vi "Find Item by Tag.vi"(8 "error in (no error)":errorcluster, 10 "Tag":string, 11 "Tree Manager in":refnum<class "Tree Manager.lvclass">) -> (0 "error out":errorcluster, 1 "Found?":bool, 2 "Data Item":refnum<class "Data Item.lvclass">, 3 "Tree Manager out":refnum<class "Tree Manager.lvclass">)   [LabVIEW 2020, in "VILab.lvlib" / "Tree Manager.lvclass"]
uses:
  Tree Manager.lvclass
  Data Item/Data Item.lvclass
  Tree Manager.lvclass/Tree Manager.ctl
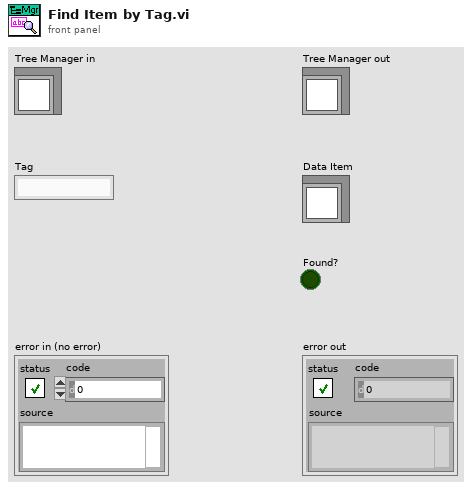
[diagram p1: front panel]
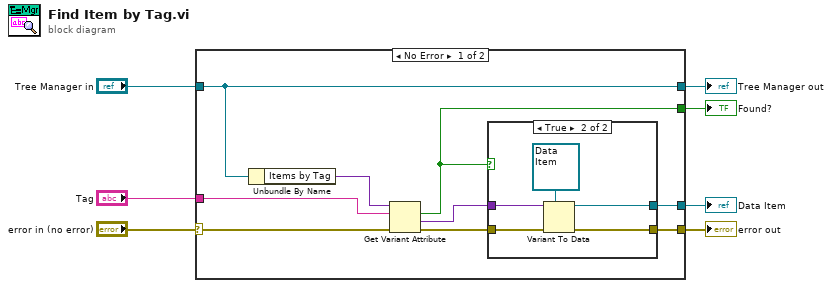
[diagram p0: block diagram]
diagram:
  n1 = case shown="No Error" "error in (no error)" {
    selector: "error in (no error)" -> [w13 w24]
    tunnel: [w10 w24] -> w6
    tunnel: [w16 w23] -> w4
    tunnel: "Tree Manager in" -> [w16 w23]
    tunnel: "Tag" -> [w14 _]
    tunnel: [w8 _] -> w2
    tunnel: [w11 _] -> w1
    frame No Error {
      n2 = Unbundle By Name(w16) -> ("Items by Tag"=w15:variant)
      n3 = Get Variant Attribute(Variant=w15, name=w14, error in=w13) -> (found=w8:bool, value=w9:variant, error out=w12:errorcluster)  [unwired: 1 in, 1 out]
      n4 = case shown="True" w8 {
        tunnel: w9 -> [_ w22]
        tunnel: w12 -> [w17 w20]
        tunnel: [_ w19] -> w11
        tunnel: [w17 w18] -> w10
        frame False {
        }
        frame True {
          n5 = Variant To Data(error in=w20, type=refnum<class "Data Item.lvclass"> refnum ("VILab.lvlib:Data Item.lvclass"), Variant=w22) -> (data=w19:refnum<class "Data Item.lvclass">, error out=w18:errorcluster)
        }
      }
    }
    frame Error {
    }
  }
  "error out" <- w6
  "Tree Manager out" <- w4
  "Found?" <- w2
  "Data Item" <- w1
